vi "Write Timestamp Configuration.vi"(8 "error in (no error)":errorcluster, 9 "Value":timestamp, 10 "Name":string, 11 "database-configuration in":refnum<class "configuration-database.lvclass">) -> (0 "error out":errorcluster, 3 "database-configuration out":refnum<class "configuration-database.lvclass">)   [LabVIEW 2020, in "configuration-database.lvlib" / "configuration-database.lvclass"]
uses:
  configuration-database.lvclass
  configuration-database.lvclass/configuration-database.ctl
  702f793f-0d20-4190-aab1-46d76a2f4f1c.vi
  <vilib>/Utility/error.llb/Error Cluster From Error Code.vi
  IConfigDBQueries/IConfigurationDatabaseQueries.lvclass
  externals/database-interface/IDatabase/IDatabase/IDatabase.lvclass
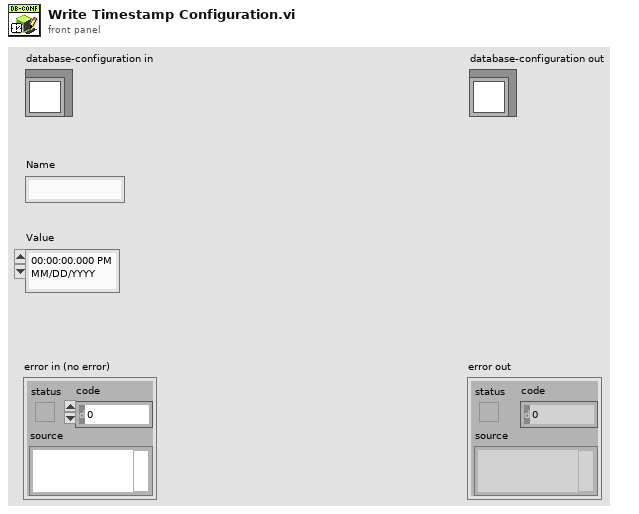
[diagram p1: front panel]
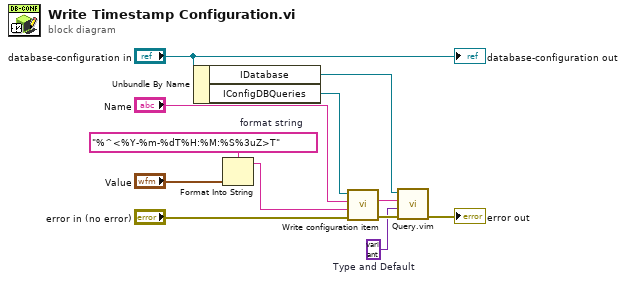
[diagram p0: block diagram]
diagram:
  w1 = variant  # Type and Default
  w7 = "%^<%Y-%m-%dT%H:%M:%S%3uZ>T"  # format string
  n1 = Unbundle By Name("database-configuration in") -> ("IDatabase"=w4:refnum<class "IDatabase.lvclass">, "IConfigDBQueries"=w12:refnum<class "IConfigurationDatabaseQueries.lvclass">)
  n2 = Format Into String(format string=w7, "Value") -> (resulting string=w5:string)  [unwired: 2 in, 1 out]
  n3 = call-dynamic "Write configuration item.vi"("error in (no error)"="error in (no error)", "Value"=w5, "Name in"="Name", "IConfigDBQueries in"=w12) -> ("error out"=w2:errorcluster, "Query"=w3:string)  [unwired: 6 in]
  n4 = call "Query.vim"("error in (no error)"=w2, "Type and Default"=w1, "Query string"=w3, "IDatabase in"=w4) -> ("error out"=→"error out":errorcluster)  [unwired: 5 in, 2 out]
  "database-configuration out" <- "database-configuration in"
